vi "Pre Launch Init.vi"(11 "VisionUI in":refnum<class "VisionUI.lvclass">) -> (0 "error out":errorcluster, 3 "VisionUI out":refnum<class "VisionUI.lvclass">)   [LabVIEW 2019, in "VisionUI.lvlib" / "VisionUI.lvclass"]
doc: "(<B>Filename</B>: Actor Framework.lvlib:Actor.lvclass:Pre Launch Init.vi)\n\nDefines behavior that occurs after the Launch Nested Actor method is invoked but before the actor's Actor Core method begins running.\n\nBy default, this method does nothing. A descendant class may override it to define behavior."
uses:
  VisionUI.lvclass
  <vilib>/vision/Image Controls.llb/IMAQ Image.ctl
  VisionUI.lvclass/VisionUI.ctl
  SubVI/SaveAsync.vi
  Vision/Vision/Vision.lvclass
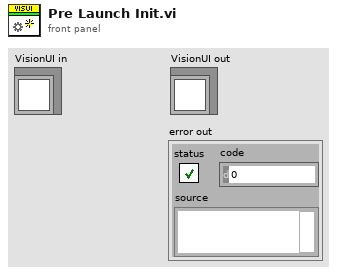
[diagram p1: front panel]
types:
  T1 = typedef "IMAQ Image.ctl" = refnum<image>
  T2 = cluster{"stop":refnum<user-event>, "Image":refnum<user-event>, "Extracts":refnum<user-event>, "UI":refnum<user-event>}
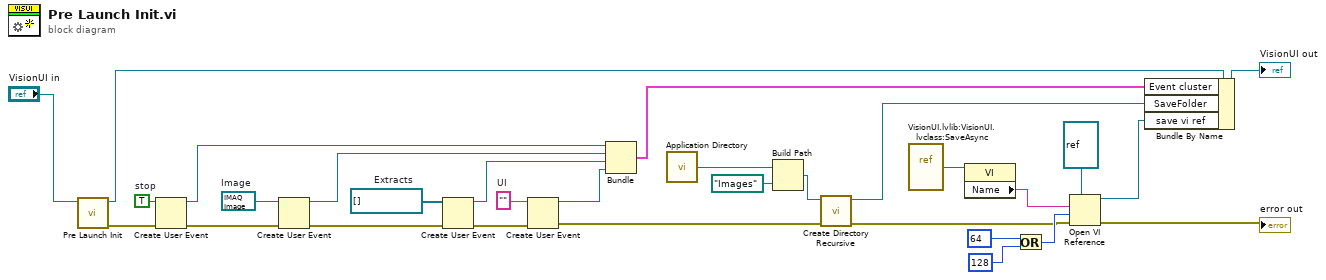
[diagram p0: block diagram]
diagram:
  w16 = ""  # UI
  w20 = T1[] []  # Extracts
  w25 = T1 refnum  # Image
  w28 = TRUE  # stop
  n1 = call-parent "Pre Launch Init.vi"("Vision in"="VisionUI in") -> ("error out"=w27:errorcluster, "Vision out"=w30:refnum<class "VisionUI.lvclass">)  [unwired: 9 in]
  n2 = Create User Event(user event datatype=w28, error in=w27) -> (user event=w22:refnum<user-event>, error out=w24:errorcluster)
  n3 = Create User Event(user event datatype=w25, error in=w24) -> (user event=w23:refnum<user-event>, error out=w19:errorcluster)
  n4 = Create User Event(user event datatype=w20, error in=w19) -> (user event=w18:refnum<user-event>, error out=w17:errorcluster)
  n5 = Create User Event(user event datatype=w16, error in=w17) -> (user event=w15:refnum<user-event>, error out=w11:errorcluster)
  n6 = Bundle("stop"=w22, "Image"=w23, "Extracts"=w18, "UI"=w15) -> (w21:T2)  [unwired: 1 in]
  n7 = call <vilib>:"Application Directory.vi"() -> ("Application Directory"=w14:path)
  n8 = Build Path(base path=w14, name or relative path=path "Images") -> (appended path=w12:path)
  n9 = call <vilib>:"Create Directory Recursive.vi"("error in (no error)"=w11, "directory"=w12) -> ("error out"=w3:errorcluster, "directory copy"=w10:path)  [unwired: 3 in, 1 out]
  n10 = vi-ref "VisionUI.lvlib:VisionUI.lvclass:SaveAsync.vi"() -> (w8:refnum<vi>)
  n11 = property class="VI"(reference=w8) -> ("Name"=w7:string)  [unwired: 1 in, 2 out]
  n12 = Or(x=64, y=128) -> (x .or. y?=w4:i32)
  n13 = Open VI Reference(type specifier VI Refnum (for type only)=refnum<vi> refnum, vi path=w7, options=w4, error in (no error)=w3) -> (vi reference=w1:refnum<vi>, error out=→"error out":errorcluster)  [unwired: 2 in]
  n14 = Bundle By Name(cluster=w30, "Event cluster"=w21, "SaveFolder"=w10, "save vi ref"=w1) -> (→"VisionUI out":refnum<class "VisionUI.lvclass">)
